vi "email warning.vi"(8 "Message":string="Error or timeout in ", 9 "running VI":string="Wait_for_Temp.vi", 10 "Initial":timestamp=timestamp(3580924707.4018655 s since 1904-01-01), 11 "email interval (min)":dbl) -> (0 "notified timestamp":timestamp)   [LabVIEW 2020]
panel:
  out "elapsed time (s)":dbl
  out "error out":errorcluster
  in  "error in (no error)":errorcluster
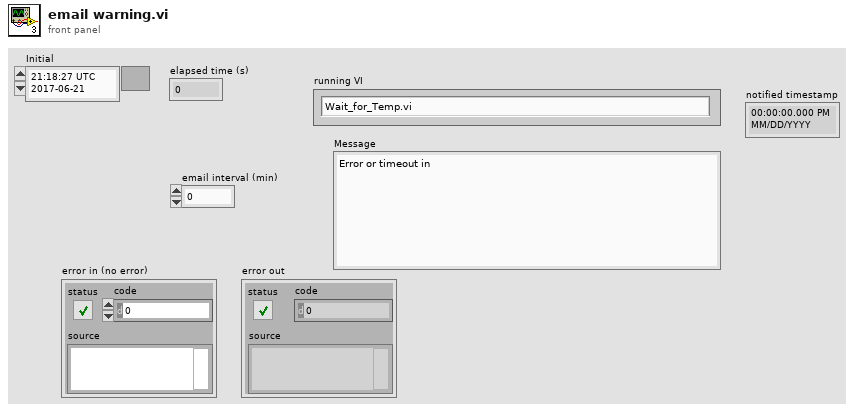
[diagram p1: front panel]
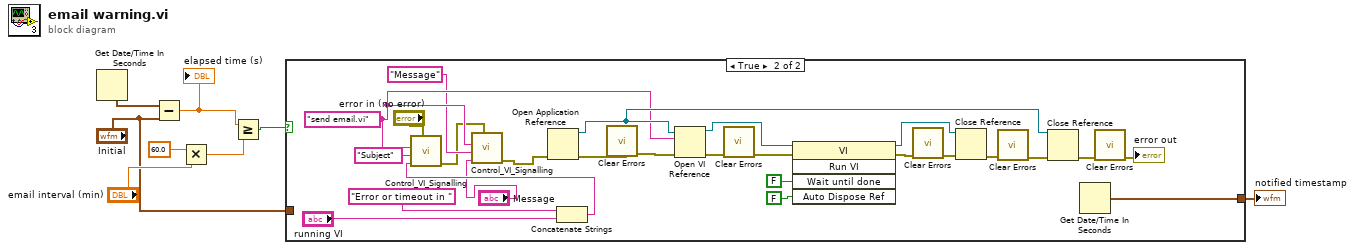
[diagram p0: block diagram]
diagram:
  n1 = Get Date/Time In Seconds() -> (seconds since 1Jan1904=w8:timestamp)
  n2 = Subtract(x=w8, y="Initial") -> (x-y=w7:dbl)
  "elapsed time (s)" <- w7
  n3 = Multiply(x=60.0, y="email interval (min)") -> (x*y=w4:dbl)
  n4 = Greater Or Equal?(x=w7, y=w4) -> (x >= y?=w3:bool)
  n5 = case shown="True" w3 {
    tunnel: [w9 w15] -> w1
    tunnel: "Initial" -> [w9 _]
    frame False {
    }
    frame True {
      w13 = "send email.vi" ("Target VI name")
      n6 = Concatenate Strings("Error or timeout in ", "running VI") -> (w16:string)
      n7 = call "Control_VI_Signalling.vi"("error in (no error)"="error in (no error)", "Input Value"=w16, "Control Name"="Subject", "Target VI name"=w13) -> ("error out"=w11:errorcluster)  [unwired: 7 in]
      n8 = call "Control_VI_Signalling.vi"("error in (no error)"=w11, "Input Value"="Message", "Control Name"="Message", "Target VI name"=w13) -> ("error out"=w14:errorcluster)  [unwired: 7 in]
      n9 = Open Application Reference(8:w14) -> (0:w27:errorcluster, 3:w26:refnum<vi>)  [unwired: 3 in]
      n10 = call <vilib>:"Clear Errors.vi"("error in (no error)"=w27) -> ("error out"=w28:errorcluster)  [unwired: 5 in, 1 out]
      n11 = Open VI Reference(application reference (local)=w26, vi path=w13, error in (no error)=w28) -> (vi reference=w22:refnum<vi>, error out=w29:errorcluster)  [unwired: 3 in]
      n12 = call <vilib>:"Clear Errors.vi"("error in (no error)"=w29) -> ("error out"=w30:errorcluster)  [unwired: 5 in, 1 out]
      n13 = invoke class="VI" method="Run VI"(reference=w22, error in=w30, "Wait until done"=FALSE ("Wait Until Done"), "Auto Dispose Ref"=FALSE ("Auto Dispose Reference")) -> (reference out=w25:refnum<vi>, error out=w31:errorcluster)  [unwired: 1 in, 3 out]
      n14 = call <vilib>:"Clear Errors.vi"("error in (no error)"=w31) -> ("error out"=w32:errorcluster)  [unwired: 5 in, 1 out]
      n15 = Close Reference(reference=w25, error in (no error)=w32) -> (error out=w33:errorcluster)
      n16 = call <vilib>:"Clear Errors.vi"("error in (no error)"=w33) -> ("error out"=w34:errorcluster)  [unwired: 5 in, 1 out]
      n17 = Close Reference(reference=w26, error in (no error)=w34) -> (error out=w35:errorcluster)
      n18 = Get Date/Time In Seconds() -> (seconds since 1Jan1904=w15:timestamp)
      n19 = call <vilib>:"Clear Errors.vi"("error in (no error)"=w35) -> ("error out"=→"error out":errorcluster)  [unwired: 5 in, 1 out]
    }
  }
  "notified timestamp" <- w1
